vi "SetPersistentConfiguration.vi"(8 "Error In":errorcluster, 9 "DataIn":variant, 11 "reference in":refnum<class "UserManager.lvclass">) -> (0 "Error Out":errorcluster, 1 "DataOut":variant, 3 "reference out":refnum<class "UserManager.lvclass">)   [LabVIEW 2021, in "UserMananger.lvlib" / "UserManager.lvclass"]
uses:
  UserManager.lvclass
  a2d9dd7e-4f73-47a2-b010-087cab1955c7.vi
  <vilib>/Utility/LVClass/Get LV Class Name.vi
  Library_TAF_ApplicationFramework/TAFBaseGUI/TAFBaseGUI.lvclass
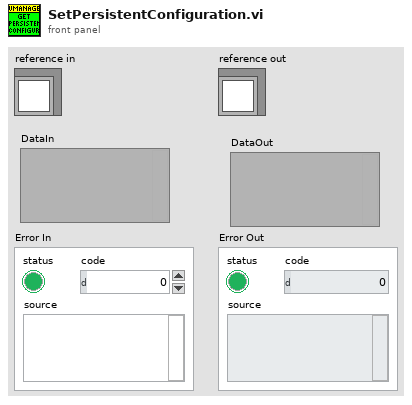
[diagram p1: front panel]
types:
  T1 = typedef "UserMananger.lvlib/UserManager.lvclass/ObjectAttributes.ctl" = cluster{"Interfaces":cluster{"ActivationUpdated":refnum<class "IAuthorizationUpdated.lvclass">}, "Locals":cluster{"MainGUIActive":refnum<queue>, "Evaluations":cluster{"Label":string, "Value":string}[]}, "Persistent":cluster{"Dummy":bool}}
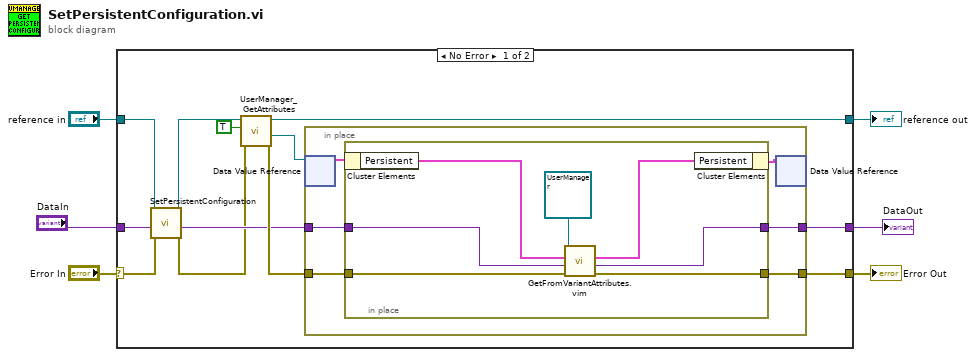
[diagram p0: block diagram]
diagram:
  n1 = case shown="No Error" "Error In" {
    selector: "Error In" -> [w8 w34]
    tunnel: [w17 w34] -> w5
    tunnel: [w16 w33] -> w3
    tunnel: "reference in" -> [w9 w33]
    tunnel: [w15 w32] -> w2
    tunnel: "DataIn" -> [w11 w32]
    frame No Error {
      n2 = call-parent "SetPersistentConfiguration.vi"("Error In"=w8, "DataIn"=w11, "reference in"=w9) -> ("Error Out"=w7:errorcluster, "DataOut"=w12:variant, "reference out"=w10:refnum<class "UserManager.lvclass">)  [unwired: 6 in]
      n3 = call "UserManager_GetAttributes.vi"("error in (no error)"=w7, "OnlyGetDvrReference(False)"=TRUE, "reference in"=w10) -> ("error out"=w18:errorcluster, "DataRef"=w13:refnum<data-value>, "reference out"=w16:refnum<class "UserManager.lvclass">)  [unwired: 5 in, 1 out]
      n4 = in-place {
        in-place-border: w18 -> [w24]
        in-place-border: [w23] -> w17
        in-place-border: w12 -> [w22]
        in-place-border: [w21] -> w15
        n5 = in-place-dvr #1(w13) -> (w20:T1)  [unwired: 1 out]
        n6 = in-place {
          in-place-border: w24 -> [w31]
          in-place-border: [w25] -> w23
          in-place-border: w22 -> [w30]
          in-place-border: [w29] -> w21
          n7 = in-place-cluster #2(w20) -> ("Persistent"=w27:cluster{"Dummy":bool})
          n8 = call "GetFromVariantAttributes.vim"("error in (no error)"=w31, "DataIn in"=w30, "PersistentDataType"=w27, "Object"=refnum<class "UserManager.lvclass"> refnum ("VerticalButtonBar")) -> ("error out"=w25:errorcluster, "Data out"=w29:variant, "PersistentDataOut"=w26:cluster{"Dummy":bool})  [unwired: 5 in]
          n9 = in-place-cluster #2("Persistent"=w26) -> (w19:T1)
        }
        n10 = in-place-dvr #1(w19) -> ()  [unwired: 2 out]
      }
    }
    frame Error {
    }
  }
  "Error Out" <- w5
  "reference out" <- w3
  "DataOut" <- w2
